vi "Centimeter To Pixels.vi"(1 "PPI":i32, 2 "CM":dbl) -> (0 "Pixels":dbl)   [LabVIEW 2019]
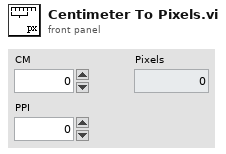
[diagram p1: front panel]
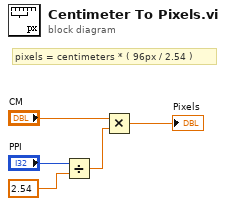
[diagram p0: block diagram]
diagram:
  # "pixels = centimeters * ( 96px / 2.54 )"
  n1 = Divide(x="PPI", y=2.54) -> (x/y=w2:dbl)
  n2 = Multiply(x="CM", y=w2) -> (x*y=→"Pixels":dbl)
